vi "Draw_Base.vi"(10 "last two points":cluster{dbl, dbl}[](array[cluster]), 11 "picture in":picture) -> (2 "wireframe":picture, 3 "picture out":picture)   [LabVIEW 2022 SP3]
uses:
  Perspective_Globals.vi
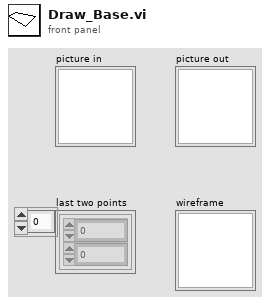
[diagram p1: front panel]
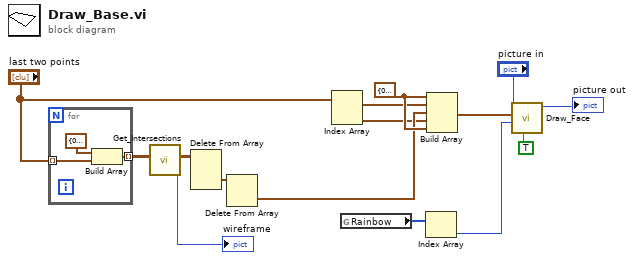
[diagram p0: block diagram]
diagram:
  w6 = cluster{dbl, dbl} {0.0, 0.0}
  n1 = for {
    tunnel: "last two points" -> [w18] mode=indexing
    tunnel: [w16] -> w13 mode=indexing
    n2 = Build Array(cluster{dbl, dbl} {0.0, 0.0}, w18) -> (w16:cluster{dbl, dbl}[])
  }
  n3 = call "Get_Intersections.vi"("Edge Points"=w13) -> ("All Points"=w15:cluster{"x":dbl, "y":dbl}[][], "picture out"=→"wireframe":picture)  [unwired: 9 in]
  n4 = Delete From Array(array=w15) -> (deleted portion=w2:cluster{"x":dbl, "y":dbl}[])  [unwired: 3 in, 1 out]
  n5 = Delete From Array(array=w2) -> (deleted portion=w5:cluster{"x":dbl, "y":dbl})  [unwired: 2 in, 1 out]
  n6 = Index Array(array="last two points") -> (element #1=w3:cluster{dbl, dbl}, element #2=w4:cluster{dbl, dbl})  [unwired: 2 in]
  n7 = global read "Perspective_Globals.vi" "Rainbow"() -> (w1:u32[])
  n8 = Index Array(array=w1) -> (element=w9:u32)  [unwired: 1 in]
  n9 = Build Array(w6, w3, w5, w4, w6) -> (w7:cluster{"x":dbl, "y":dbl}[])
  n10 = call "Draw_Face.vi"("fill?(F)"=TRUE, "color"=w9, "Array"=w7, "picture in"="picture in") -> ("new picture"=→"picture out":picture)  [unwired: 7 in]
